vi "33.vi"() -> ()   [LabVIEW 2019]
uses:
  <vilib>/MakerHub/LINX/LMH-LINX.lvlib
  <vilib>/MakerHub/LINX/Public/Utilities/Open Serial.vi
  <vilib>/MakerHub/LINX/Public/Sensors/Motion/Servo/Servo.lvlib
  <vilib>/MakerHub/LINX/Public/Sensors/Motion/Servo/Servo Set Pulse Width One Channel.vi
  <vilib>/MakerHub/LINX/Public/Sensors/Motion/Servo/Servo Open One Channel.vi
  <vilib>/addons/control/pid/NI_PID_pid.lvlib
  <vilib>/addons/control/pid/pid.llb/PID (DBL).vi
  <vilib>/MakerHub/LINX/Public/Sensors/Motion/Servo/Servo Close One Channel.vi
  <vilib>/MakerHub/LINX/Public/Peripherals/Analog/Analog Read 1 Chan.vi
panel:
  out "output 2":dbl(graph)=1897.9601723247413
  in  "Analog Channel":u8=1
  out "output":dbl=1897.9601723247413 format="%.2f"
  out "dt out (s)":dbl=0.009000000427477062 format="%.3f"
  in  "PID gains":T1={"proportional gain (Kc)"=3.8, "integral time (Ti, min)"=0.038, "derivative time (Td, min)"=0.002} {"derivative time (Td, min)" format="%.3f"; "integral time (Ti, min)" format="%.3f"; "proportional gain (Kc)" format="%.3f"}
  in  "dt (s)":dbl=-1.0 format="%.3f"
  in  "output range":cluster{"output high":dbl, "output low":dbl}={"output high"=2200.0, "output low"=1400.0} {"output low" format="%.2f"; "output high" format="%.2f"}
  in  "reinitialize? (F)":bool
  in  "setpoint":dbl=2.9 format="%.2f"
  in  "Servo Channel":u8=9
  in  "Serial Port":refnum<visa-resource-name>="COM7"
  in  "stop":bool
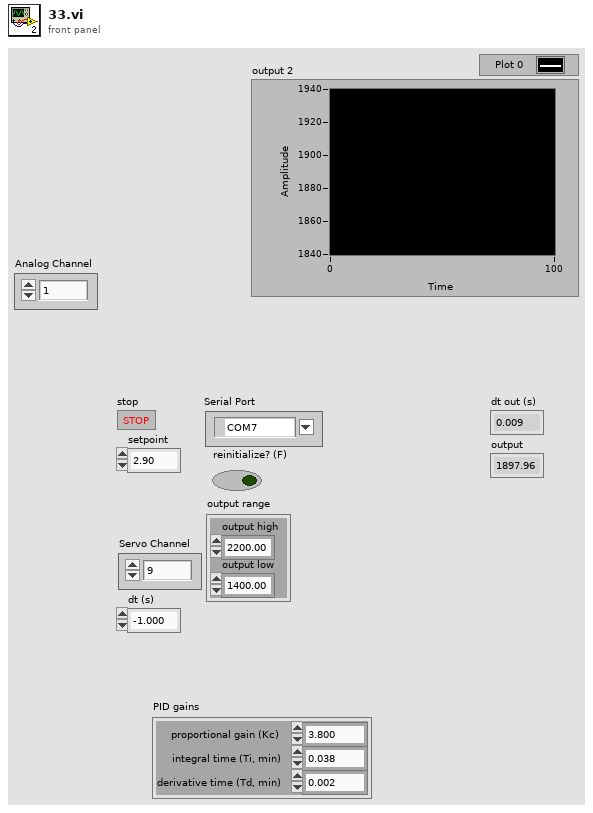
[diagram p1: front panel]
types:
  T1 = cluster{"proportional gain (Kc)":dbl, "integral time (Ti, min)":dbl, "derivative time (Td, min)":dbl}
  T2 = typedef "LMH-LINX.lvlib/LINX Ref.ctl" = cluster{"IO":T3, "Interface":T4, "LINX Device Config":T5}
  T3 = typedef "LMH-LINX.lvlib/Platform.ctl" = enum16{"Remote", "Local"}
  T4 = typedef "LMH-LINX.lvlib/Interface.ctl" = enum16{"Serial", "TCP"}
  T5 = typedef "LMH-LINX.lvlib/Device.lvlib/LINX Device Config.ctl" = cluster{"Interface":T4, "COM Port":refnum<visa-resource-name>, "TCP Configuration":T6, "Device Family":u8, "Device ID":u8, "Device Name":string, "TCP Ref":refnum<k5>, "Channels":T7}
  T6 = typedef "LMH-LINX.lvlib/Device.lvlib/TCP Config.ctl" = cluster{"IP Address":string, "Port":u16}
  T7 = typedef "LMH-LINX.lvlib/Channels.ctl" = cluster{"DI":u8[], "DO":u8[], "AI":u8[], "AO":u8[], "PWM":u8[], "QE":u8[], "UART":u8[], "I2C 2":u8[], "SPI":u8[], "CAN":u8[], "Servo":u8[], "AI Ref (V)":dbl, "AI Resolution (Bits)":u8, "AO Ref (V)":dbl, "AO Resolution (Bits)":u8}
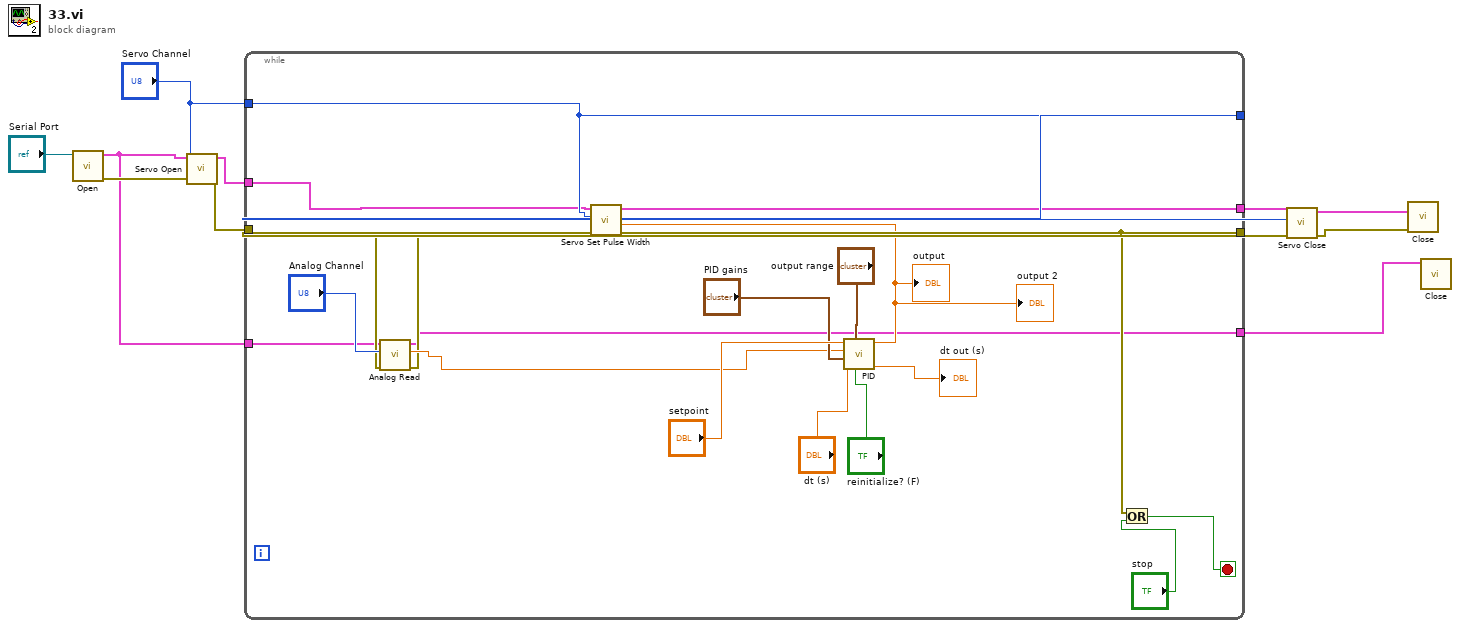
[diagram p0: block diagram]
diagram:
  n1 = call-poly <vilib>:"Open.vi"("Serial Port"="Serial Port") -> ("Error Out"=w3:errorcluster, "LINX Resource"=w2:T2)  [unwired: 8 in, 1 out]
  n2 = call-poly <vilib>:"Servo Open.vi"("Error In"=w3, "Servo Channel"="Servo Channel", "LINX Resource"=w2) -> ("Error Out"=w8:errorcluster, "LINX Resource"=w9:T2)  [unwired: 7 in]
  n3 = while {
    tunnel: [w14] -> w12
    tunnel: [w30] -> w11
    tunnel: w9 -> [w16]
    tunnel: w8 -> [w18]
    tunnel: "Servo Channel" -> [w28]
    tunnel: [w28] -> w6
    tunnel: w2 -> [w15]
    tunnel: [w13] -> w1
    stop <- w29 stop-if-true
    n4 = call-poly <vilib>:"Analog Read.vi"("Error In"=w18, "Analog Channel"="Analog Channel", "LINX Resource"=w15) -> ("Error Out"=w17:errorcluster, "Voltage"=w19:dbl, "LINX Resource"=w13:T2)  [unwired: 5 in, 1 out]
    n5 = call-poly <vilib>:"PID.vi"("reinitialize? (F)"="reinitialize? (F)", "output range"="output range", "dt (s)"="dt (s)", "PID gains"="PID gains", "process variable"=w19, "setpoint"="setpoint") -> ("dt out (s)"=→"dt out (s)":dbl, "output"=w21:dbl)  [unwired: 4 in]
    "output" <- w21
    "output 2" <- w21
    n6 = call-poly <vilib>:"Servo Set Pulse Width.vi"("Error In"=w17, "Pulse Width (uS)"=w21, "Servo Channel"=w28, "LINX Resource"=w16) -> ("Error Out"=w30:errorcluster, "LINX Resource"=w14:T2)  [unwired: 6 in]
    n7 = Or(x=w30, y="stop") -> (x .or. y?=w29:bool)
  }
  n8 = call-poly <vilib>:"Servo Close.vi"("Error In"=w11, "Servo Channel"=w6, "LINX Resource"=w12) -> ("Error Out"=w5:errorcluster, "LINX Resource"=w10:T2)  [unwired: 7 in]
  n9 = call <vilib>:"Close.vi"("Error In"=w5, "LINX Resource"=w10) -> ()  [unwired: 9 in, 1 out]
  n10 = call <vilib>:"Close.vi"("LINX Resource"=w1) -> ()  [unwired: 10 in, 1 out]
